vi "test_contrast_map.vi"() -> ()   [LabVIEW 2009]
doc: "Copyright (C) 2009, Stepan A. Baranov\nweb: http://www.OCTLab.org/\nemail: stepan@baranov.su"
uses:
  <vilib>/Analysis/NI_AALBase.lvlib
  OCTLib.dll
panel:
  out "version":string
  out "name":string
  out "error out":errorcluster
  out "radius":i32
  out "width":i32
  out "height":i32
  in  "Small/Big":bool
  out "loop #":i32
  out "RSM_STAT time":u32
  out "LabView time":u32
  out "RSM_STAT Array":dbl[][](array[numeric])
  out "LabView Array":dbl[][](array[numeric])
  in  "stop":bool
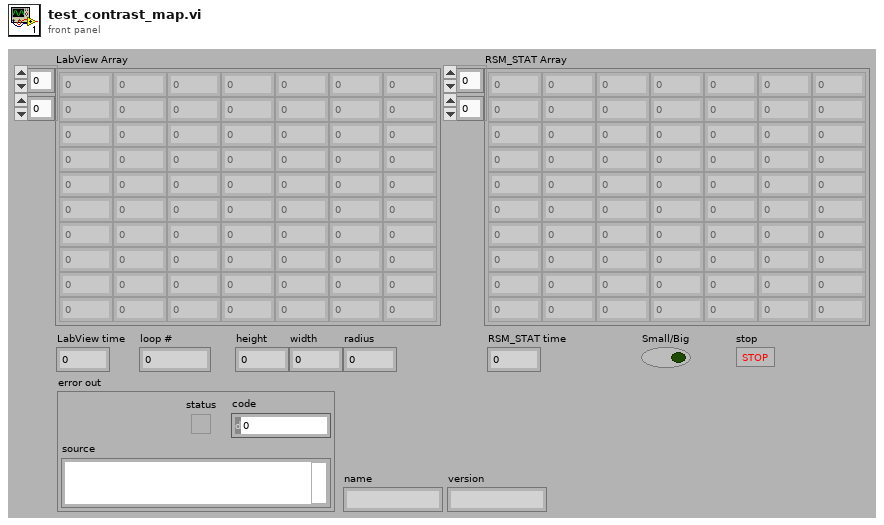
[diagram p1: front panel]
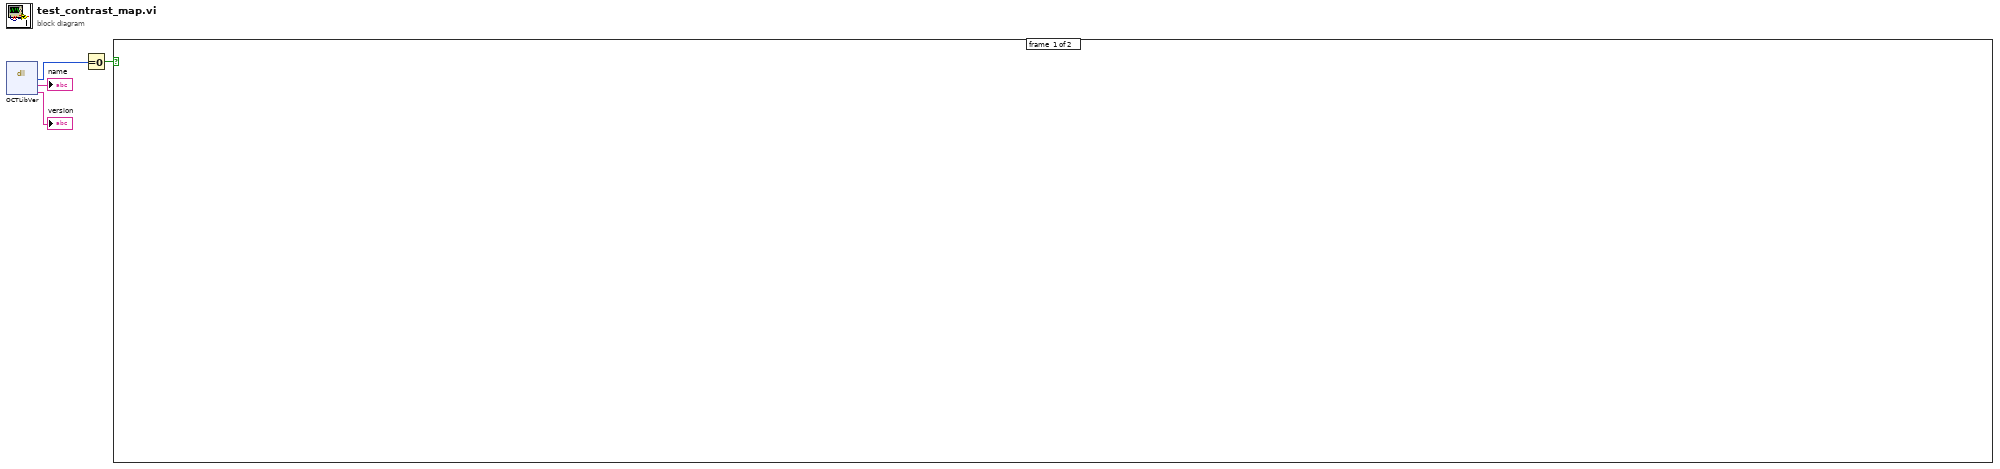
[diagram p0: block diagram]
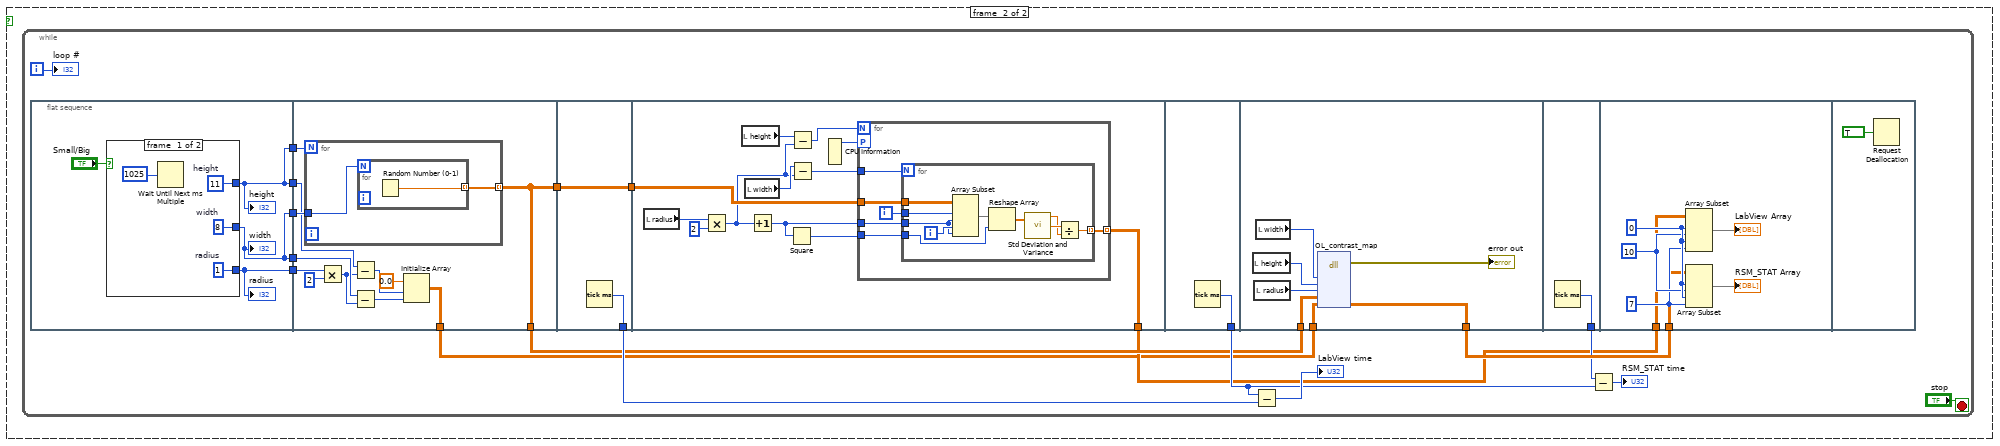
[diagram p2: hidden frame]
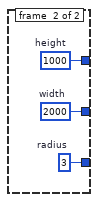
[diagram p3: hidden frame]
diagram:
  n1 = dll-call lib="OCTLib.dll" fn="OCTLibVer"() -> ("status"=w4:i8, "name"=→"name":string, "version"=→"version":string)  [unwired: 5 in, 2 out]
  n2 = Equal To 0?(x=w4) -> (x = 0?=w1:bool)
  n3 = case shown="True" w1 {
    frame #0 {
    }
    frame #1 {
      n4 = while {
        i -> [w15]
        stop <- "stop" stop-if-true
        n5 = flat-sequence {
          tunnel: [w23] -> w11
          tunnel: [w24] -> w10
          tunnel: [w25] -> w8
          tunnel: [w24] -> w7
          tunnel: [w23] -> w6
          tunnel: [w43] -> w14
          tunnel: [w43] -> w12
          tunnel: w11 -> [w45]
          tunnel: w10 -> [w44]
          tunnel: w8 -> [w41]
          tunnel: w7 -> [w39]
          tunnel: w6 -> [w37]
          tunnel: [w34] -> w5
          tunnel: [w50] -> w20
          tunnel: [w49] -> w13
          tunnel: w12 -> [w49]
          tunnel: w13 -> [w62]
          tunnel: [w58] -> w9
          tunnel: [w79] -> w17
          tunnel: w14 -> [w85]
          tunnel: [w84] -> w21
          tunnel: w5 -> [w86]
          tunnel: [w87] -> w18
          tunnel: w21 -> [w90]
          tunnel: w9 -> [w89]
          frame #0 {
            n6 = case shown="True" "Small/Big" {
              tunnel: [w28 w33] -> w24
              tunnel: [w29 w32] -> w23
              tunnel: [w30 w31] -> w25
              frame #0 {
                w30 = 1  # radius
                w29 = 8  # width
                w28 = 11  # height
                n7 = Wait Until Next ms Multiple(millisecond multiple=u32 1025) -> ()  [unwired: 1 out]
              }
              frame #1 {
                w31 = 3  # radius
                w32 = 2000  # width
                w33 = 1000  # height
              }
            }
            "height" <- w24
            "width" <- w23
            "radius" <- w25
          }
          frame #1 {
            n8 = for {
              N: w44 -> [_]
              tunnel: w45 -> [w47]
              tunnel: [w46] -> w43 mode=indexing
              n9 = for {
                N: w47 -> [_]
                tunnel: [w48] -> w46 mode=indexing
                n10 = Random Number (0-1)() -> (number: 0 to 1=w48:dbl)
              }
            }
            n11 = Multiply(x=w41, y=2) -> (x*y=w36:i32)
            n12 = Subtract(x=w39, y=w36) -> (x-y=w38:i32)
            n13 = Subtract(x=w37, y=w36) -> (x-y=w35:i32)
            n14 = Initialize Array(0.0 ("element"), w38, w35) -> (w34:dbl[][])
          }
          frame #2 {
            n15 = Tick Count (ms)() -> (millisecond timer value=w50:u32)
          }
          frame #3 {
            n16 = local read "radius"() -> (w61:i32)
            n17 = Multiply(x=w61, y=2) -> (x*y=w53:i32)
            n18 = local read "height"() -> (w56:i32)
            n19 = local read "width"() -> (w54:i32)
            n20 = Increment(x=w53) -> (x+1=w57:i32)
            n21 = Square(x=w57) -> (x^2=w59:i32)
            n22 = Subtract(x=w56, y=w53) -> (x-y=w55:i32)
            n23 = Subtract(x=w54, y=w53) -> (x-y=w52:i32)
            n24 = CPU Information() -> (4:w51:i32)  [unwired: 3 out]
            n25 = for {
              N: w55 -> [_]
              tunnel: w62 -> [w67]
              tunnel: w59 -> [w66]
              tunnel: [w65] -> w58 mode=indexing
              tunnel: w57 -> [w64]
              tunnel: w52 -> [w63]
              workers-P: w51 -> [_]
              i -> [w68]
              n26 = for {
                N: w63 -> [_]
                tunnel: w68 -> [w78]
                tunnel: w67 -> [w76]
                tunnel: w66 -> [w72]
                tunnel: [w75] -> w65 mode=indexing
                tunnel: w64 -> [w74]
                i -> [w77]
                n27 = Array Subset(array=w76, index (row)=w78, length (row)=w74, index (col)=w77, length (col)=w74) -> (w73:dbl[][])
                n28 = Reshape Array(w73, w72) -> (w71:dbl[])
                n29 = call <vilib>:"Std Deviation and Variance.vi"("X"=w71) -> ("mean"=w69:dbl, "standard deviation"=w70:dbl)  [unwired: 1 in, 1 out]
                n30 = Divide(x=w70, y=w69) -> (x/y=w75:dbl)
              }
            }
          }
          frame #4 {
            n31 = Tick Count (ms)() -> (millisecond timer value=w79:u32)
          }
          frame #5 {
            n32 = local read "height"() -> (w82:i32)
            n33 = local read "radius"() -> (w81:i32)
            n34 = local read "width"() -> (w83:i32)
            n35 = dll-call lib="OCTLib.dll" fn="OL_contrast_map"("width"=w83, "height"=w82, "radius"=w81, "input"=w85, "output"=w86) -> (error out=→"error out":errorcluster, "output"=w84:dbl[][])  [unwired: 8 in, 1 out]
          }
          frame #6 {
            n36 = Tick Count (ms)() -> (millisecond timer value=w87:u32)
          }
          frame #7 {
            w93 = 10 ("length")
            w92 = 7 ("length")
            w94 = 0 ("index")
            n37 = Array Subset(array=w89, index (row)=w94, length (row)=w93, index (col)=w94, length (col)=w92) -> (→"LabView Array":dbl[][])
            n38 = Array Subset(array=w90, index (row)=w94, length (row)=w93, index (col)=w94, length (col)=w92) -> (→"RSM_STAT Array":dbl[][])
          }
          frame #8 {
            n39 = Request Deallocation(TRUE ("flag")) -> ()
          }
        }
        n40 = Subtract(x=w17, y=w20) -> (x-y=→"LabView time":u32)
        n41 = Subtract(x=w18, y=w17) -> (x-y=→"RSM_STAT time":u32)
        "loop #" <- w15
      }
    }
  }
